vi "TDMS In Memory Write to Network.vi"() -> ()   [LabVIEW 2023]
doc: "This example demonstrates the use of the TDMS In Memory functions to write a .tdms file in memory to the network."
panel:
  out "Waveform Graph":waveform(dbl)(graph)
  # "Overview: Demonstrates the use of the TDMS In Memory functions to write a .tdms file in memory to the network. \nInstructions:\nRun this VI. Waveform Graph displays the data of the .tdms file written to the network."
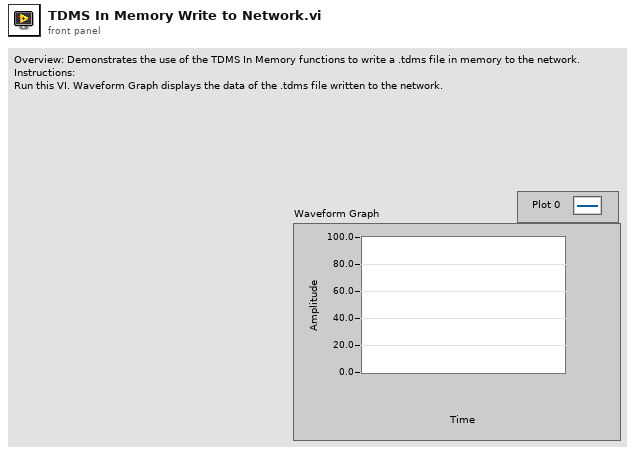
[diagram p1: front panel]
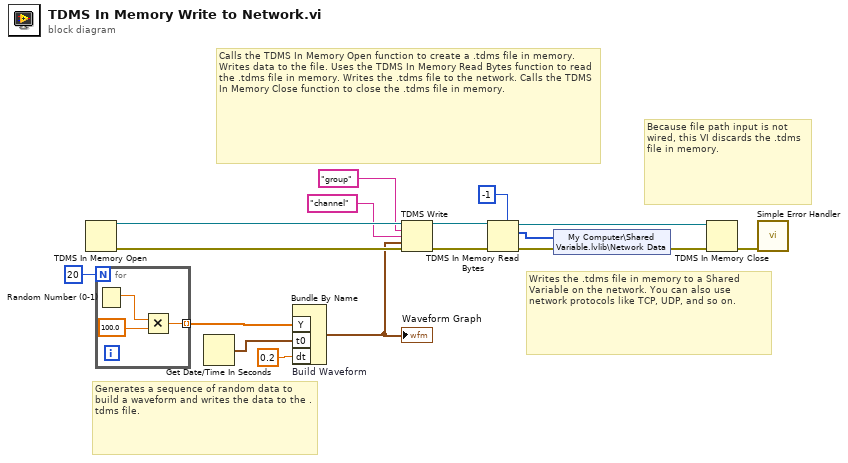
[diagram p0: block diagram]
diagram:
  # "Because file path input is not wired, this VI discards the .tdms file in memory."
  # "Generates a sequence of random data to build a waveform and writes the data to the .tdms file."
  # "Calls the TDMS In Memory Open function to create a .tdms file in memory. Writes data to the file. Uses the TDMS In Memory Read Bytes function to read the .tdms file in memory. Writes the .tdms file to the network. Calls the TDMS In Memory Close function to close the .tdms file in memory."
  # "Writes the .tdms file in memory to a Shared Variable on the network. You can also use network protocols like TCP, UDP, and so on."
  n1 = TDMS In Memory Open() -> (0:w15:errorcluster, 3:w16:refnum<k34>)  [unwired: 2 in]
  n2 = for {
    N: 20 ("# points") -> [_]
    tunnel: [w19] -> w6 mode=indexing
    n3 = Random Number (0-1)() -> (number: 0 to 1=w20:dbl)
    n4 = Multiply(x=w20, y=100.0) -> (x*y=w19:dbl)
  }
  n5 = Get Date/Time In Seconds() -> (seconds since 1Jan1904=w5:timestamp)
  n6 = Bundle By Name "Build Waveform"("Y"=w6, "t0"=w5, "dt"=0.2) -> (w1:waveform(dbl))  [unwired: 1 in]
  "Waveform Graph" <- w1
  n7 = TDMS Write(0:w16, 5:"group" ("group name in (Untitled)"), 7:"channel", 9:w1, 11:w15) -> (4:w13:refnum<k34>, 15:w11:errorcluster)  [unwired: 1 in, 2 out]
  n8 = TDMS In Memory Read Bytes(5:i64 -1 ("byte count (-1: all)"), 8:w11, 11:w13) -> (0:w9:errorcluster, 2:w2:u8[], 3:w12:refnum<k34>)  [unwired: 1 in]
  n9 = shared-variable "My Computer\\Shared Variable.lvlib\\Network Data"(w2, error in=w9) -> (error out=w8:errorcluster)
  n10 = TDMS In Memory Close(8:w8, 11:w12) -> (0:w17:errorcluster)  [unwired: 2 in]
  n11 = call <vilib>:"Simple Error Handler.vi"("error in (no error)"=w17) -> ()  [unwired: 4 in, 5 out]
